vi "ImageCreation.vi"() -> ()   [LabVIEW 2015]
panel:
  in  "Add Noise":bool
  in  "Noise":dbl=-1.0 format="%#_13g"
  out "Image Out":T1(plugin-control)
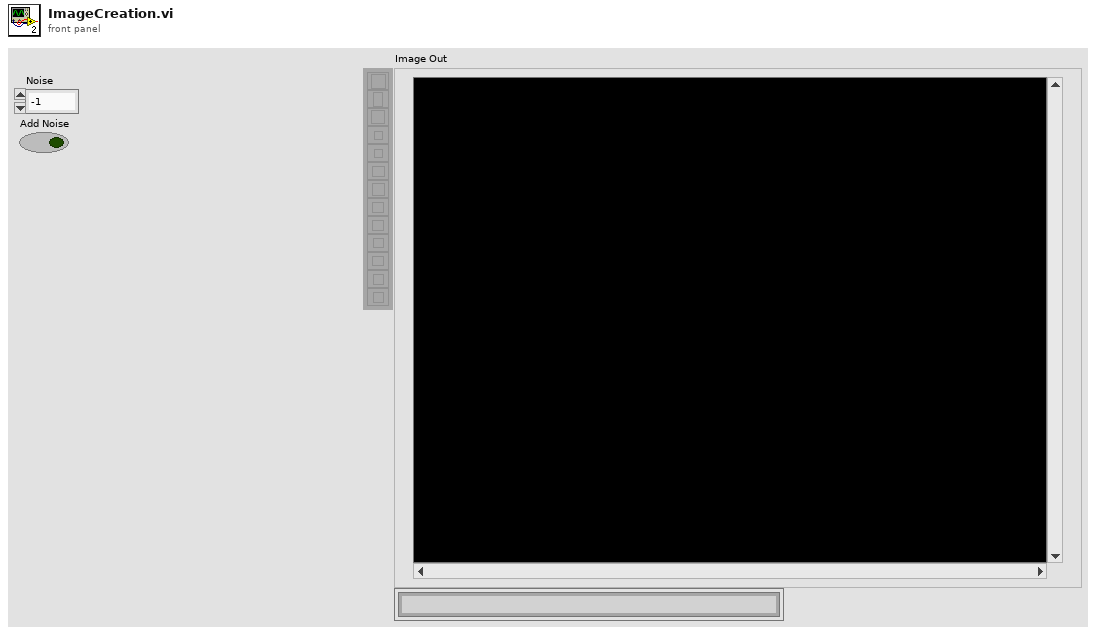
[diagram p1: front panel]
types:
  T1 = typedef "IMAQ Image.ctl" = refnum<image>
  T2 = typedef "Image Type" = u32
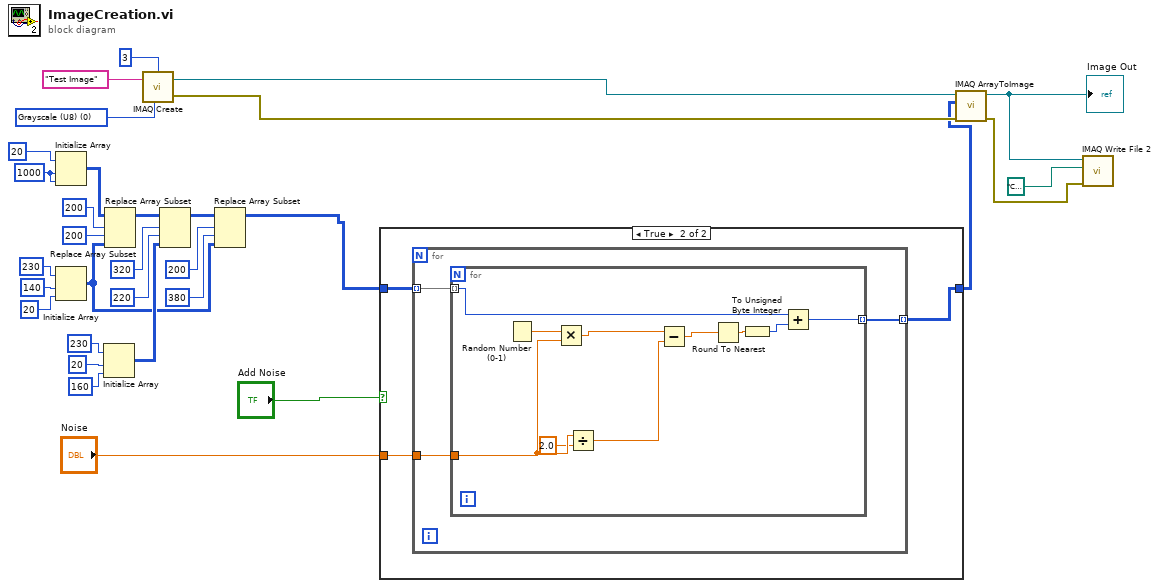
[diagram p0: block diagram]
diagram:
  w27 = 1000 ("dimension size")
  w30 = T2 0 items=["Grayscale (U8)", "Grayscale (I16)", "Grayscale (SGL)", "Complex (CSG)", "RGB (U32)", "HSL (U32)", "RGB (U64)", "Grayscale (U16)"] ("Image Type")
  n1 = Initialize Array(u8 20 ("element"), w27, w27) -> (w24:u8[][])
  n2 = Initialize Array(u8 230 ("element"), 140 ("dimension size"), 20 ("dimension size")) -> (w11:u8[][])
  n3 = Initialize Array(u8 230 ("element"), 20 ("dimension size"), 160 ("dimension size")) -> (w15:u8[][])
  n4 = Replace Array Subset(array=w24, new element=w11, index (row)=200, index (col)=200 ("disabled index (col)")) -> (w16:u8[][])
  n5 = call "IMAQ Create"("Border Size"=3, "Image Name"="Test Image", "Image Type"=w30) -> ("New Image"=w1:T1, "error out"=w26:errorcluster)  [unwired: 2 in]
  n6 = Replace Array Subset(array=w16, new element=w15, index (row)=320 ("disabled index (row)"), index (col)=220 ("disabled index (col)")) -> (w12:u8[][])
  n7 = Replace Array Subset(array=w12, new element=w11, index (row)=200 ("disabled index (row)"), index (col)=380 ("disabled index (col)")) -> (w3:u8[][])
  n8 = case shown="True" "Add Noise" {
    tunnel: w3 -> [w32 w35]
    tunnel: "Noise" -> [_ w34]
    tunnel: [w32 w33] -> w2
    frame False {
    }
    frame True {
      n9 = for {
        tunnel: w35 -> [w38] mode=indexing
        tunnel: w34 -> [w37]
        tunnel: [w36] -> w33 mode=indexing
        n10 = for {
          tunnel: w38 -> [w45] mode=indexing
          tunnel: w37 -> [w43]
          tunnel: [w44] -> w36 mode=indexing
          n11 = Random Number (0-1)() -> (number: 0 to 1=w48:dbl)
          n12 = Multiply(x=w48, y=w43) -> (x*y=w41:dbl)
          n13 = Divide(x=w43, y=2.0) -> (x/y=w40:dbl)
          n14 = Subtract(x=w41, y=w40) -> (x-y=w39:dbl)
          n15 = Round To Nearest(number=w39) -> (nearest integer value=w47:dbl)
          n16 = To Unsigned Byte Integer(number=w47) -> (unsigned 8bit integer=w46:u8)
          n17 = Add(x=w45, y=w46) -> (x+y=w44:u8)
        }
      }
    }
  }
  n18 = call "IMAQ ArrayToImage"("error in (no error)"=w26, "Image Pixels (U8)"=w2, "Image"=w1) -> ("error out"=w6:errorcluster, "Image Out"=w8:T1)  [unwired: 7 in]
  "Image Out" <- w8
  n19 = call-poly "IMAQ Write File 2"("error in (no error)"=w6, "File Path"=path "C:/Users/Admin/Documents/TestImage.png", "Image"=w8) -> ()  [unwired: 7 in, 2 out]
